vi "Get Section.vi"(10 "Section":string, 11 "EDS in":refnum<class "EDS.lvclass">) -> (1 "Found?":bool, 2 "Section":refnum<class "Section.lvclass">, 3 "EDS out":refnum<class "EDS.lvclass">)   [LabVIEW 2024]
uses:
  EDS/EDS.lvclass
  OD Section/Section.lvclass
  Object Dictionary/Dictionary.lvclass
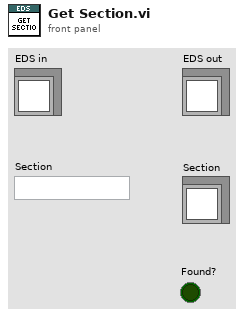
[diagram p1: front panel]
types:
  T1 = typedef "EDS.lvclass/ObjectAttributes.ctl" = cluster{"EDS File Path":path, "Object Dict":refnum<class "Dictionary.lvclass">, "Sorted Object Dict":refnum<class "Sorted Object Dictionary.lvclass">, "Device Info":refnum<class "Device Info.lvclass">, "File Info":refnum<class "File Info.lvclass">}
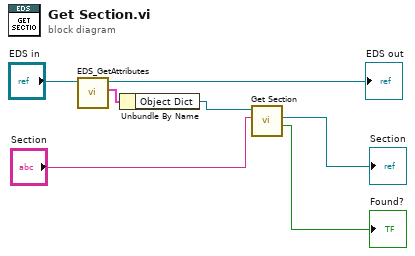
[diagram p0: block diagram]
diagram:
  n1 = call "EDS_GetAttributes.vi"("reference in"="EDS in") -> ("Data"=w2:T1, "reference out"=→"EDS out":refnum<class "EDS.lvclass">)  [unwired: 7 in, 2 out]
  n2 = Unbundle By Name(w2) -> ("Object Dict"=w1:refnum<class "Dictionary.lvclass">)
  n3 = call "Get Section.vi"("Section"="Section", "Dictionary in"=w1) -> ("Found?"=→"Found?":bool, "Section out"=→"Section":refnum<class "Section.lvclass">)  [unwired: 7 in, 1 out]
